vi "RDV-addDataToGraph.vi"(8 "error in (no error)":errorcluster, 11 "RDV-Reflection_Data_viewer in":refnum<class "RDV-Reflection_Data_viewer.lvclass">) -> (0 "error out":errorcluster, 3 "RDV-Reflection_Data_viewer out":refnum<class "RDV-Reflection_Data_viewer.lvclass">)   [LabVIEW 2020, in "RDV-Reflection_Data_viewer.lvclass"]
uses:
  RDV-Reflection_Data_viewer.lvclass
  RDV-Reflection_Data_viewer.lvclass/RDV-Reflection_Data_viewer.ctl
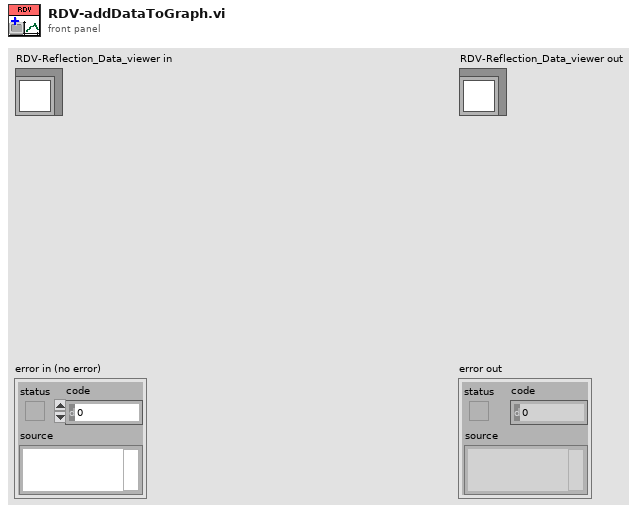
[diagram p1: front panel]
types:
  T1 = typedef "RDV-Reflection_Data_viewer.lvclass/RDV-XY_GRAPH_REFS.ctl" = cluster{"Reflection Real":refnum<vi>, "Reflection Imag":refnum<vi>, "Permittivity Real":refnum<vi>, "Permittivity Imag":refnum<vi>}
  T2 = cluster{"Frequency":dbl[], "Reflection'":dbl[]}[]
  T3 = cluster{"Frequency":dbl[], "Reflection'":dbl[]}[][]
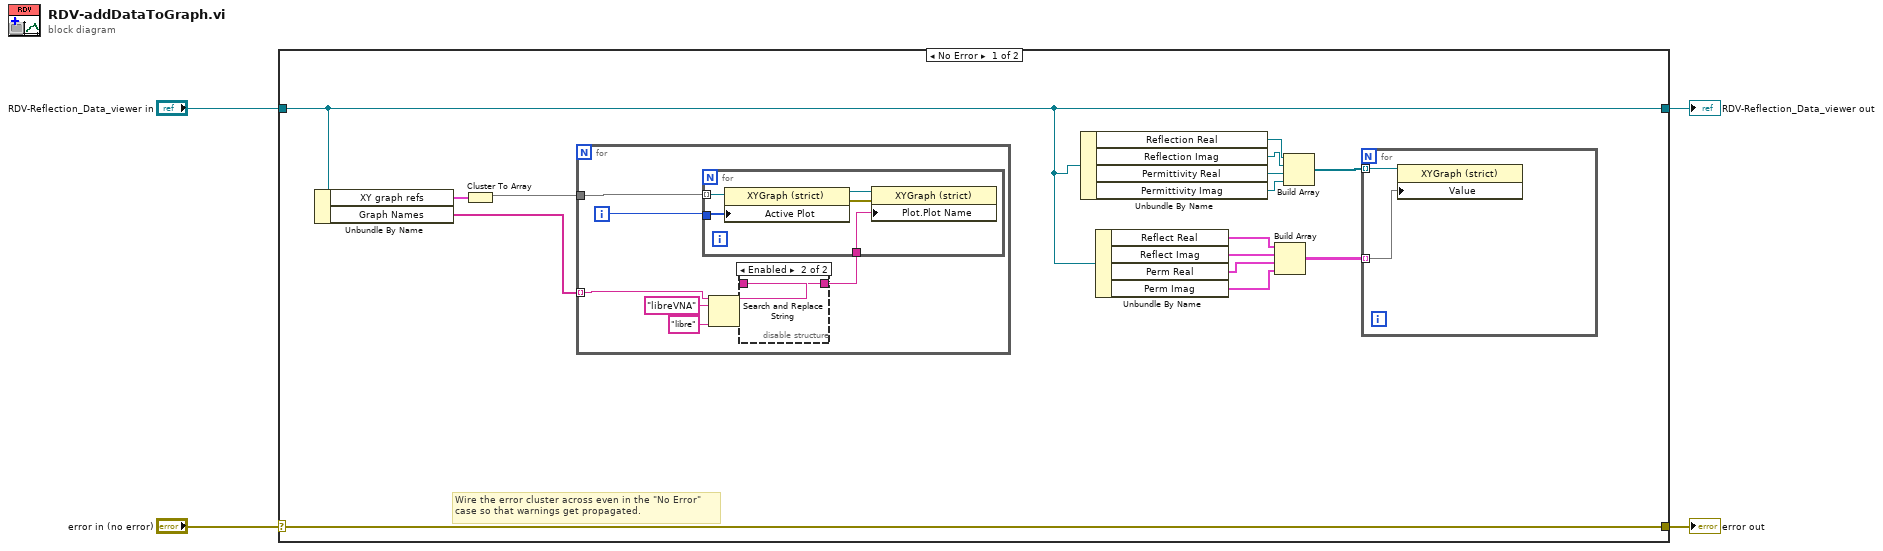
[diagram p0: block diagram]
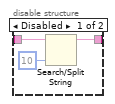
[diagram p2: hidden frame]
diagram:
  n1 = case shown="No Error" "error in (no error)" {
    selector: "error in (no error)" -> [w19 w39]
    tunnel: [w19 w39] -> w3
    tunnel: [w11 w38] -> w1
    tunnel: "RDV-Reflection_Data_viewer in" -> [w11 w38]
    frame No Error {
      # "Wire the error cluster across even in the \"No Error\"\ncase so that warnings get propagated."
      n2 = Unbundle By Name(w11) -> ("XY graph refs"=w17:T1, "Graph Names"=w18:string[])
      n3 = Cluster To Array(cluster=w17) -> (array=w12:refnum<vi>[])
      n4 = for {
        tunnel: w12 -> [w21]
        tunnel: w18 -> [w20] mode=indexing
        i -> [w26]
        n5 = Search and Replace String(input string=w20, search string="libreVNA", replace string="libre" ("replace string (\"\")")) -> (result string=w22:string)  [unwired: 5 in, 3 out]
        n6 = disable-structure shown="Enabled" {
          disable-tunnel: [w28 w30] -> w25
          disable-tunnel: w22 -> [w27 w30]
          frame Disabled {
            n7 = Search/Split String(string=w27, offset (0)=10) -> (substring before match=w28:string)  [unwired: 1 in, 2 out]
          }
          frame Enabled {
          }
        }
        n8 = for {
          tunnel: w26 -> [w35]
          tunnel: w25 -> [w34]
          tunnel: w21 -> [w33] mode=indexing
          n9 = property on="Property Node" class="XYGraph (strict)"(reference=w33, "Active Plot"=w35) -> (reference out=w32:refnum<vi>, error out=w31:errorcluster)  [unwired: 1 in]
          n10 = property on="Property Node" class="XYGraph (strict)"(reference=w32, error in=w31, "Plot.Plot Name"=w34) -> ()  [unwired: 2 out]
        }
      }
      n11 = Unbundle By Name(w11) -> ("Reflection Real"=w10:refnum<vi>, "Reflection Imag"=w9:refnum<vi>, "Permittivity Real"=w8:refnum<vi>, "Permittivity Imag"=w7:refnum<vi>)
      n12 = Unbundle By Name(w11) -> ("Reflect Real"=w16:T2, "Reflect Imag"=w15:T2, "Perm Real"=w14:T2, "Perm Imag"=w13:T2)
      n13 = Build Array(w16, w15, w14, w13) -> (w5:T3)
      n14 = Build Array(w10, w9, w8, w7) -> (w6:refnum<vi>[])
      n15 = for {
        tunnel: w6 -> [w37] mode=indexing
        tunnel: w5 -> [w36] mode=indexing
        n16 = property on="Property Node" class="XYGraph (strict)"(reference=w37, "Value"=w36) -> ()  [unwired: 1 in, 2 out]
      }
    }
    frame Error {
    }
  }
  "error out" <- w3
  "RDV-Reflection_Data_viewer out" <- w1
